vi "Create.vi"(8 "error in (no error)":errorcluster, 11 "Database Manager":refnum<class "Database Manager.lvclass">) -> (0 "error out":errorcluster, 3 "Objects out":refnum<class "Objects.lvclass">)   [LabVIEW 2019, in "HierDAL Library.lvlib" / "Database.lvlib" / "Repositories.lvlib" / "Objects.lvclass"]
uses:
  Objects.lvclass
  Database Manager Class/Database Manager.lvclass
  Objects.lvclass/Objects.ctl
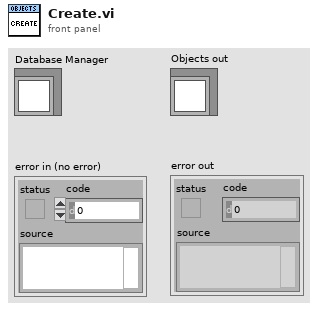
[diagram p1: front panel]
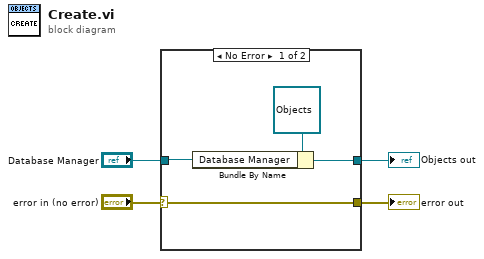
[diagram p0: block diagram]
diagram:
  n1 = case shown="No Error" "error in (no error)" {
    selector: "error in (no error)" -> [w8 w9]
    tunnel: [w8 w9] -> w3
    tunnel: [w5 _] -> w2
    tunnel: "Database Manager" -> [w6 _]
    frame No Error {
      n2 = Bundle By Name(cluster=refnum<class "Objects.lvclass"> refnum ("HierDAL Library.lvlib:Database.lvlib:Repositories.lvlib:Objects.lvclass"), "Database Manager"=w6) -> (w5:refnum<class "Objects.lvclass">)
    }
    frame Error {
    }
  }
  "error out" <- w3
  "Objects out" <- w2
